vi "ST_parse_start_operation_response.vi"(6 "recordset_in":variant[][](array[variant]), 7 "Part exists?":bool, 8 "error_in":errorcluster, 11 "command_nmb":u8) -> (0 "error_out":errorcluster, 1 "user_ID":string, 2 "save_operation_to_SQL":bool, 3 "reference_data_to_PLC":u8[](array[numeric]))   [LabVIEW 2020]
uses:
  _misc/AULocalize/SubVIs/Get Localized Phrase Compact Interface 0D.vi
  <vilib>/addons/database/_DB Variant To Data/Database Variant To Data.xnode
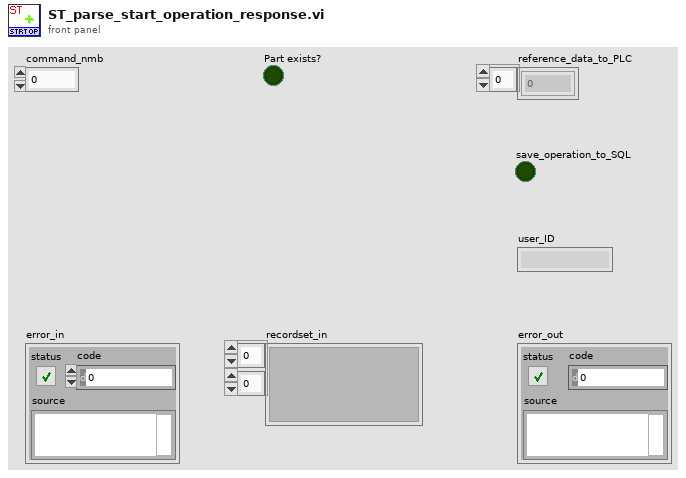
[diagram p1: front panel]
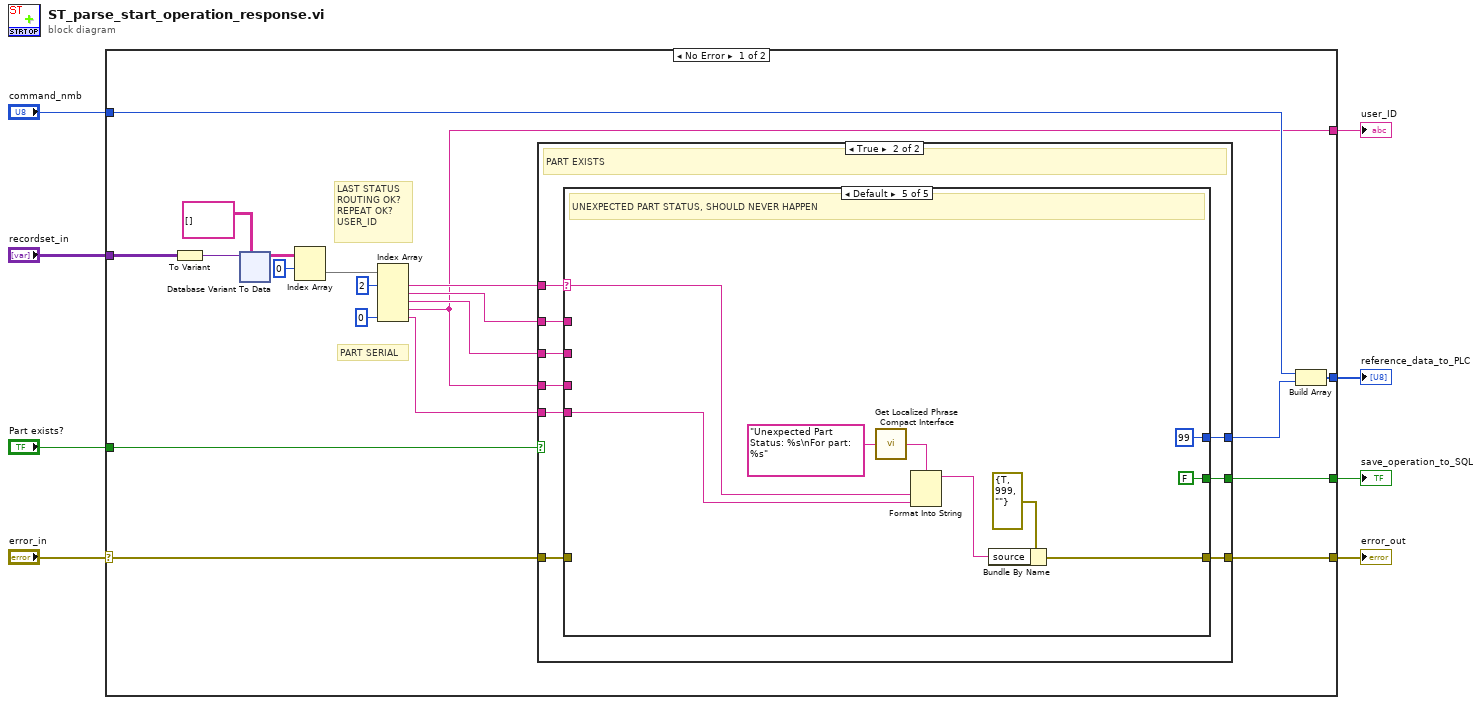
[diagram p0: block diagram]
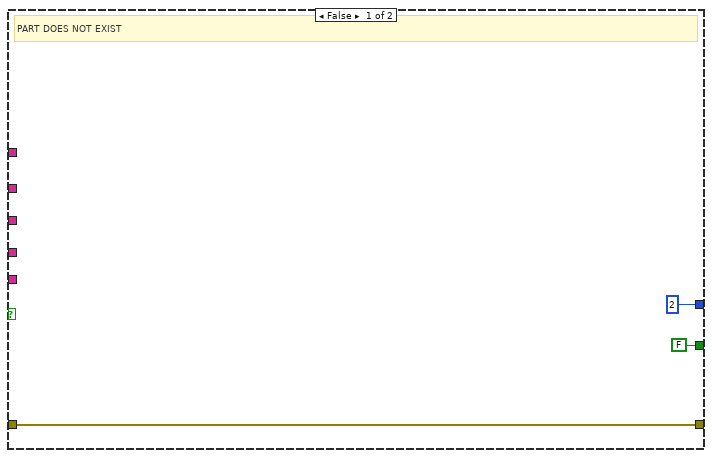
[diagram p2: hidden frame]
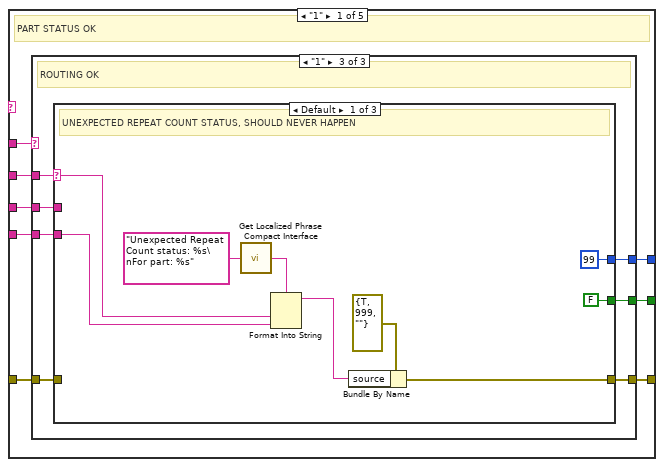
[diagram p3: hidden frame]
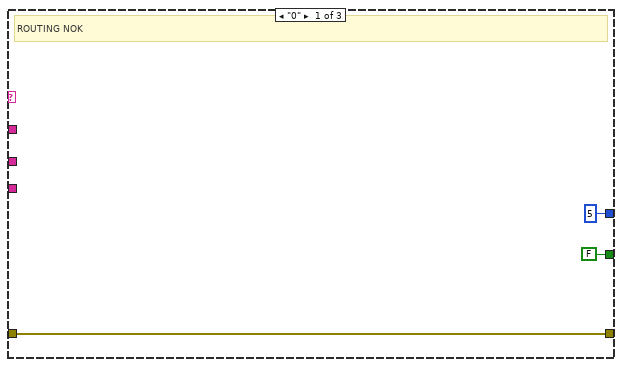
[diagram p4: hidden frame]
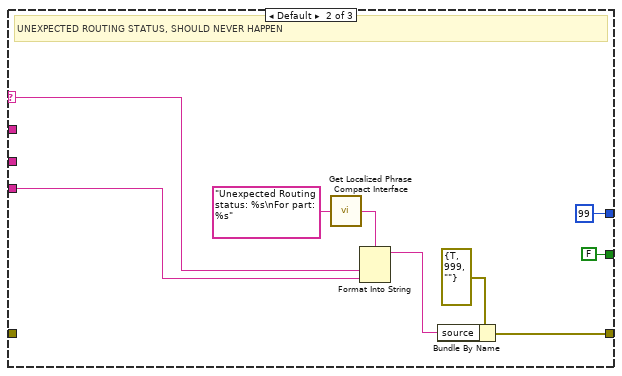
[diagram p5: hidden frame]
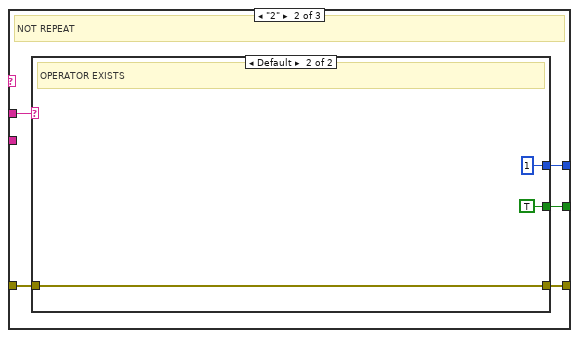
[diagram p6: hidden frame]
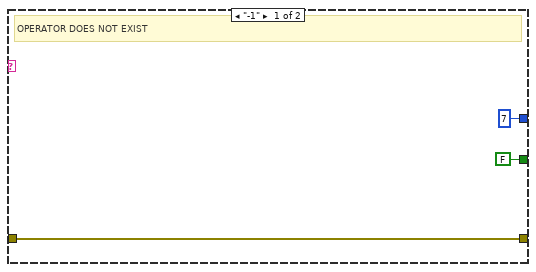
[diagram p7: hidden frame]
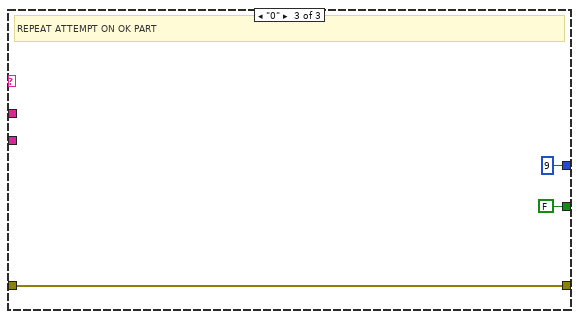
[diagram p8: hidden frame]
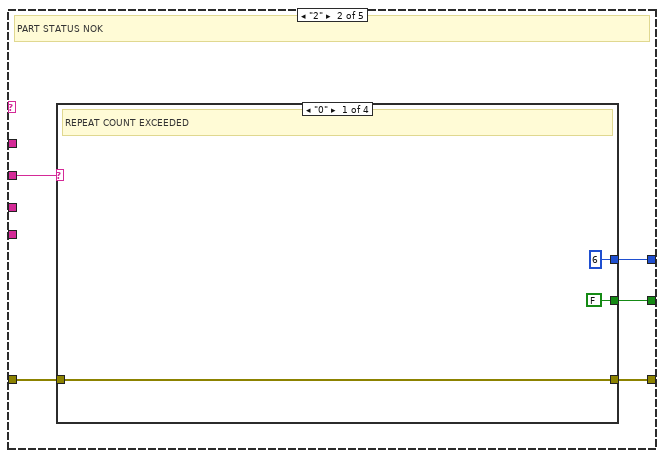
[diagram p9: hidden frame]
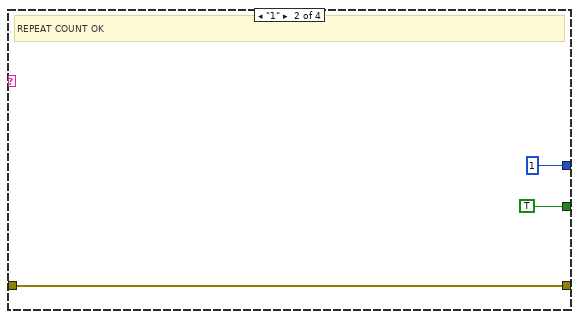
[diagram p10: hidden frame]
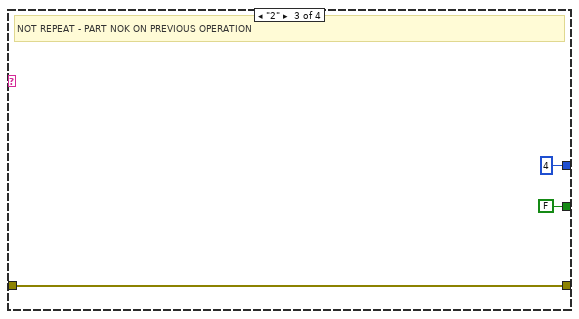
[diagram p11: hidden frame]
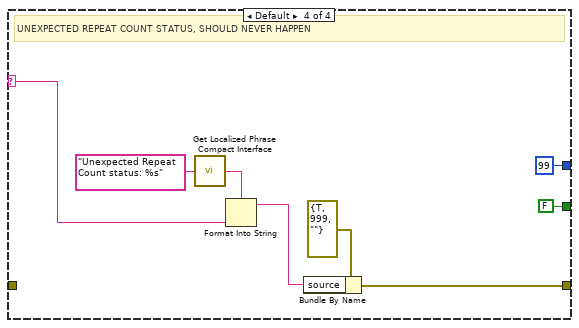
[diagram p12: hidden frame]
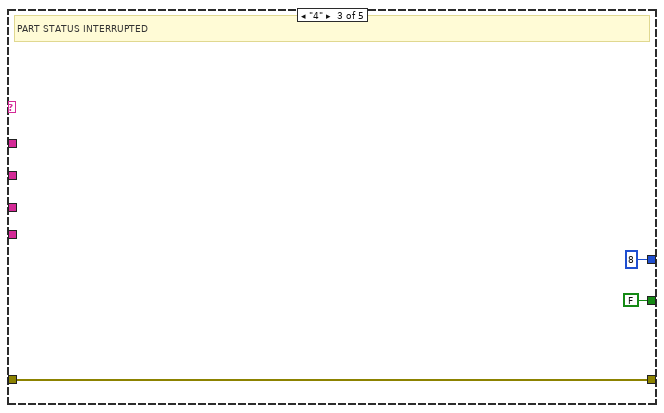
[diagram p13: hidden frame]
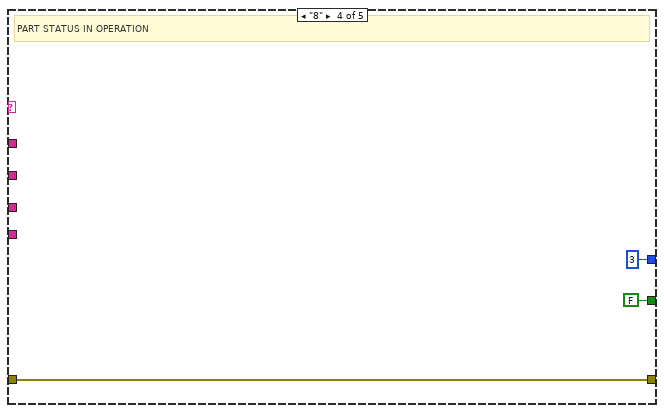
[diagram p14: hidden frame]
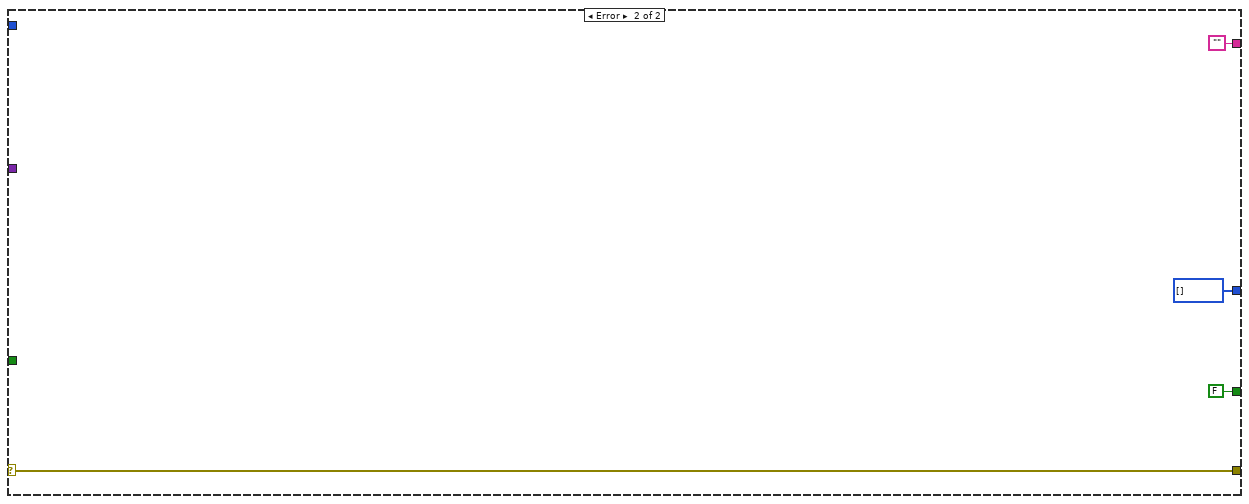
[diagram p15: hidden frame]
diagram:
  n1 = case shown="No Error" "error_in" {
    selector: "error_in" -> [w18 w163]
    tunnel: [w28 u8[] []] -> w3
    tunnel: "command_nmb" -> [w27 _]
    tunnel: "recordset_in" -> [w25 _]
    tunnel: [w17 w163] -> w5
    tunnel: [w13 FALSE] -> w4
    tunnel: [w10 ""] -> w2
    tunnel: "Part exists?" -> [w9 _]
    frame No Error {
      # "PART SERIAL"
      # "LAST STATUS\nROUTING OK?\nREPEAT OK?\nUSER_ID"
      n2 = To Variant(anything=w25) -> (Variant=w24:variant)
      n3 = xnode "Database Variant To Data"("database variant"=w24, "type"=string[][] []) -> ("data"=w23:string[][])  [unwired: 1 in, 1 out]
      n4 = Index Array(array=w23, index (row)=0) -> (element=w21:string[])  [unwired: 1 in]
      n5 = Index Array(array=w21, index #1=2 ("index"), index #5=0 ("index")) -> (element #1=w19:string, element #2=w16:string, element #3=w15:string, element #4=w10:string, element #5=w11:string)  [unwired: 3 in]
      n6 = case shown="True" w9 {
        tunnel: [u8 2 w71] -> w14
        tunnel: w19 -> [_ w72]
        tunnel: w18 -> [w62 w70]
        tunnel: [w62 w69] -> w17
        tunnel: w16 -> [_ w68]
        tunnel: w15 -> [_ w67]
        tunnel: w11 -> [_ w66]
        tunnel: [FALSE w65] -> w13
        tunnel: w10 -> [_ w64]
        frame False {
          # "PART DOES NOT EXIST"
        }
        frame True {
          # "PART EXISTS"
          n7 = case shown="Default" w72 {
            selector: w72 -> [_ _ _ _ w155]
            tunnel: [w77 w124 u8 8 u8 3 u8 99] -> w71
            tunnel: w70 -> [w79 w127 w146 w149 _]
            tunnel: [w76 w126 w146 w149 w153] -> w69
            tunnel: w68 -> [w80 _ _ _ _]
            tunnel: w67 -> [w78 w123 _ _ _]
            tunnel: w66 -> [w75 _ _ _ w154]
            tunnel: [w74 w125 FALSE FALSE FALSE] -> w65
            tunnel: w64 -> [w73 _ _ _ _]
            frame "1" {
              # "PART STATUS OK"
              n8 = case shown="\"1\"" w80 {
                selector: w80 -> [_ w87 _]
                tunnel: w79 -> [w82 _ w97]
                tunnel: w78 -> [_ _ w99]
                tunnel: [u8 5 u8 99 w98] -> w77
                tunnel: [w82 w88 w96] -> w76
                tunnel: w75 -> [_ w86 w95]
                tunnel: [FALSE FALSE w94] -> w74
                tunnel: w73 -> [_ _ w93]
                frame "0" {
                  # "ROUTING NOK"
                }
                frame Default {
                  # "UNEXPECTED ROUTING STATUS, SHOULD NEVER HAPPEN"
                  n9 = call-poly "Get Localized Phrase Compact Interface.vi"("Key"="Unexpected Routing status: %s\nFor part: %s" ("format string")) -> ("Translated Phrase"=w84:string)
                  n10 = Format Into String(format string=w84, w87, w86) -> (resulting string=w89:string)  [unwired: 2 in, 1 out]
                  n11 = Bundle By Name(cluster=errorcluster {"status"=TRUE, "code"=999, "source"=""} ("error_in"), "source"=w89) -> (w88:errorcluster)
                }
                frame "1" {
                  # "ROUTING OK"
                  n12 = case shown="Default" w99 {
                    selector: w99 -> [w103 _ _]
                    tunnel: [u8 99 w113 u8 9] -> w98
                    tunnel: w97 -> [_ w111 w121]
                    tunnel: [w106 w110 w121] -> w96
                    tunnel: w95 -> [w102 _ _]
                    tunnel: [FALSE w112 FALSE] -> w94
                    tunnel: w93 -> [_ w109 _]
                    frame Default {
                      # "UNEXPECTED REPEAT COUNT STATUS, SHOULD NEVER HAPPEN"
                      n13 = call-poly "Get Localized Phrase Compact Interface.vi"("Key"="Unexpected Repeat Count status: %s\nFor part: %s" ("format string")) -> ("Translated Phrase"=w100:string)
                      n14 = Format Into String(format string=w100, w103, w102) -> (resulting string=w104:string)  [unwired: 2 in, 1 out]
                      n15 = Bundle By Name(cluster=errorcluster {"status"=TRUE, "code"=999, "source"=""} ("error_in"), "source"=w104) -> (w106:errorcluster)
                    }
                    frame "2" {
                      # "NOT REPEAT"
                      n16 = case shown="Default" w109 {
                        tunnel: [u8 7 u8 1] -> w113
                        tunnel: [FALSE TRUE] -> w112
                        tunnel: w111 -> [w116 w117]
                        tunnel: [w116 w117] -> w110
                        frame "-1" {
                          # "OPERATOR DOES NOT EXIST"
                        }
                        frame Default {
                          # "OPERATOR EXISTS"
                        }
                      }
                    }
                    frame "0" {
                      # "REPEAT ATTEMPT ON OK PART"
                    }
                  }
                }
              }
            }
            frame "2" {
              # "PART STATUS NOK"
              n17 = case shown="\"0\"" w123 {
                selector: w123 -> [_ _ _ w140]
                tunnel: w127 -> [w128 w132 w135 _]
                tunnel: [w128 w132 w135 w143] -> w126
                tunnel: [FALSE TRUE FALSE FALSE] -> w125
                tunnel: [u8 6 u8 1 u8 4 u8 99] -> w124
                frame "0" {
                  # "REPEAT COUNT EXCEEDED"
                }
                frame "1" {
                  # "REPEAT COUNT OK"
                }
                frame "2" {
                  # "NOT REPEAT - PART NOK ON PREVIOUS OPERATION"
                }
                frame Default {
                  # "UNEXPECTED REPEAT COUNT STATUS, SHOULD NEVER HAPPEN"
                  n18 = call-poly "Get Localized Phrase Compact Interface.vi"("Key"="Unexpected Repeat Count status: %s" ("format string")) -> ("Translated Phrase"=w137:string)
                  n19 = Format Into String(format string=w137, w140) -> (resulting string=w141:string)  [unwired: 2 in, 1 out]
                  n20 = Bundle By Name(cluster=errorcluster {"status"=TRUE, "code"=999, "source"=""} ("error_in"), "source"=w141) -> (w143:errorcluster)
                }
              }
            }
            frame "4" {
              # "PART STATUS INTERRUPTED"
            }
            frame "8" {
              # "PART STATUS IN OPERATION"
            }
            frame Default {
              # "UNEXPECTED PART STATUS, SHOULD NEVER HAPPEN"
              n21 = call-poly "Get Localized Phrase Compact Interface.vi"("Key"="Unexpected Part Status: %s\nFor part: %s" ("format string")) -> ("Translated Phrase"=w151:string)
              n22 = Format Into String(format string=w151, w155, w154) -> (resulting string=w156:string)  [unwired: 2 in, 1 out]
              n23 = Bundle By Name(cluster=errorcluster {"status"=TRUE, "code"=999, "source"=""} ("error_in"), "source"=w156) -> (w153:errorcluster)
            }
          }
        }
      }
      n24 = Build Array(w27, w14) -> (w28:u8[])
    }
    frame Error {
    }
  }
  "error_out" <- w5
  "reference_data_to_PLC" <- w3
  "save_operation_to_SQL" <- w4
  "user_ID" <- w2
